vi "dfd_MA_FIFO Wrapper.vi"() -> ()   [LabVIEW 2017]
uses:
  <vilib>/rvi/Emulation/niFpgaGetClockAttributes.vi
  <vilib>/rvi/Emulation/niFpgaSctlEmulationGetInTimedLoop.vi
  <vilib>/rvi/Emulation/niFpgaEmulationReportErrorSimple.vi
  <vilib>/rvi/Emulation/niFpgaEmulationIsFPGAContextNoSignature.vi
  <vilib>/rvi/errors/niFpgaSetErrorForExecOnDevCompSimple.vi
  <vilib>/rvi/eio/common/nirviEmuReportErrorAndStop.vi
  <vilib>/rvi/DataTransferAndStorage/Container/Common/niFpgaContainerGetUniqueNameForEmu.vi
  <vilib>/rvi/FIFO/Fifo_Resource/nirvififoEmulationSetSize.vi
  <vilib>/rvi/FIFO/Fifo_Resource/nirviFifoEmulationQueueMgr.vi
  <instcachedir>/0/nirviFifoEmulationQueueMgr_E5CAEC123FF24DC58D834DCA3CDAA9B5.lvgen/nirviFifoEmulationQueueMgr_E5CAEC123FF24DC58D834DCA3CDAA9B5_002.vi
  <vilib>/Utility/error.llb/Clear Errors.vi
  <vilib>/rvi/FIFO/Fifo_Resource/nirvififoEmulationCreateLock.vi
  <vilib>/rvi/Emulation/niFpgaProcessEmulError.vi
  <vilib>/rvi/FIFO/Fifo_Resource/nirvififoEmulationObtainLock.vi
  <vilib>/rvi/FIFO/Fifo_Resource/nirvififoEmulationReleaseLock.vi
  <vilib>/rvi/occurrence/nirviWaitOnOccurrenceBase.vi
  <vilib>/rvi/errors/nirviReportUnexpectedCaseInternalError.vi
  <vilib>/rvi/errors/nirviReportUnexpectedCaseInternalError (U32).vi
  <vilib>/rvi/FIFO/Fifo_Resource/nirvififoEmulationDetermineInputValidOut.vi
  <vilib>/rvi/Emulation/niFpgaCriticalErrorInLSC.vi
  <vilib>/rvi/DataTransferAndStorage/Container/XNode/niFpgaContainer.xnode
  <vilib>/rvi/FIFO/Fifo_Resource/nirvififoEmulationRead.vi
  <vilib>/rvi/FIFO/Fifo_Resource/nirvififoEmulationWrite.vi
panel:
  in  "output valid":bool
  in  "output data":fxp<+/-,32,2> format="%.31g"
  in  "ready for input":bool
  out "input valid":bool
  out "input data":fxp<+/-,16,16>
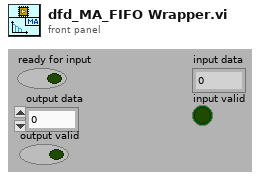
[diagram p1: front panel]
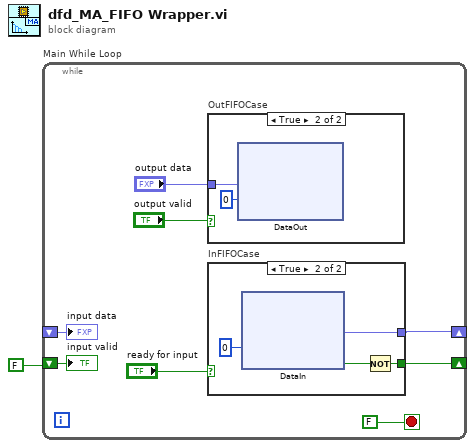
[diagram p0: block diagram]
diagram:
  n1 = while "Main While Loop" {
    shift-right: [w7] -> _
    shift-left: _ -> [w6]
    shift-right: [w9] -> _
    shift-left: FALSE ("Timed Out?") -> [w5]
    stop <- FALSE stop-if-true
    n2 = case "OutFIFOCase" shown="True" "output valid" {
      tunnel: "output data" -> [_ w11]
      frame False {
      }
      frame True {
        n3 = xnode "DataOut"("Element"=w11, "Timeout"=0) -> ()  [unwired: 1 in, 2 out]
      }
    }
    n4 = case "InFIFOCase" shown="True" "ready for input" {
      tunnel: [_ w15] -> w7
      tunnel: [_ w12] -> w9
      frame False {
      }
      frame True {
        n5 = xnode "DataIn"("Timeout"=0) -> ("Element"=w15:fxp<+/-,16,16>, "Timed Out?"=w14:bool)  [unwired: 1 in, 1 out]
        n6 = Not(x=w14) -> (.not. x?=w12:bool)
      }
    }
    "input data" <- w6
    "input valid" <- w5
  }
